vi "As PropertyObject.vi"(8 "error in (no error)":errorcluster, 11 "SequenceFile in":refnum<class "SequenceFile.lvclass">) -> (0 "error out":errorcluster, 2 "PropertyObject":refnum<k7>, 3 "SequenceFile out":refnum<class "SequenceFile.lvclass">)   [LabVIEW 2020, in "TSnax.lvlib" / "SequenceFile.lvclass"]
uses:
  SequenceFile.lvclass
  SequenceFile.lvclass/SequenceFile.ctl
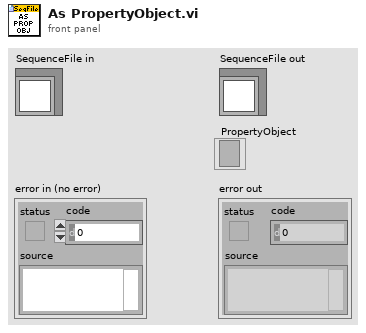
[diagram p1: front panel]
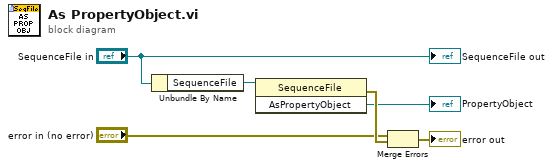
[diagram p0: block diagram]
diagram:
  n1 = Unbundle By Name("SequenceFile in") -> ("SequenceFile"=w3:refnum<k7>)
  n2 = invoke class="SequenceFile" method="AsPropertyObject"(reference=w3) -> (error out=w6:errorcluster, "AsPropertyObject"=→"PropertyObject":refnum<k7>)  [unwired: 2 in, 1 out]
  n3 = Merge Errors("error in (no error)", w6) -> (→"error out":errorcluster)
  "SequenceFile out" <- "SequenceFile in"
